vi "Is in Packed Library.vi"(8 "error in (no error)":errorcluster) -> (0 "error out":errorcluster, 3 "Is In Packed Library":bool)   [LabVIEW 2026, in "TALOS.lvlib"]
uses:
  TALOS.lvlib
  Global Memory.vi
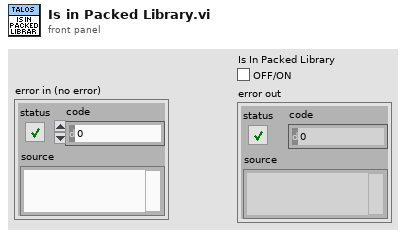
[diagram p1: front panel]
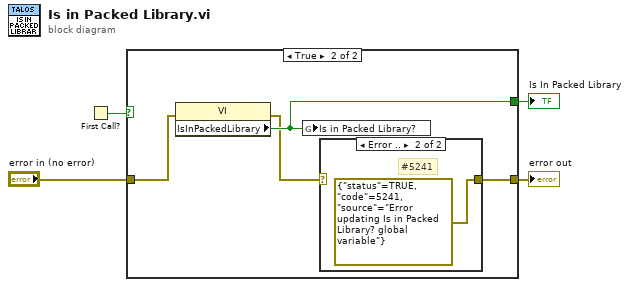
[diagram p0: block diagram]
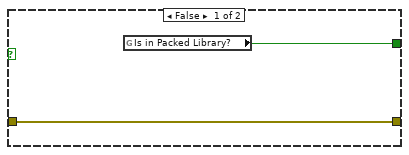
[diagram p2: hidden frame]
diagram:
  n1 = First Call?() -> (First Call?: T/F=w3:bool)
  n2 = case shown="True" w3 {
    tunnel: [w6 w10] -> w4
    tunnel: [w5 w7] -> w2
    tunnel: "error in (no error)" -> [w5 w9]
    frame False {
      n3 = global read "Global Memory.vi" "Is in Packed Library?"() -> (w6:bool)
    }
    frame True {
      n4 = property class="VI"(error in=w9) -> (error out=w8:errorcluster, "IsInPackedLibrary"=w10:bool)  [unwired: 1 in, 1 out]
      n5 = global write "Global Memory.vi" "Is in Packed Library?"(w10) -> ()
      n6 = case shown="Error .." w8 {
        selector: w8 -> [w11 _]
        tunnel: [w11 errorcluster {"status"=TRUE, "code"=5241, "source"="Error updating Is in Packed Library? global variable"} ("error IO")] -> w7
        frame No Error {
        }
        frame Error {
          # "#5241"
        }
      }
    }
  }
  "Is In Packed Library" <- w4
  "error out" <- w2
